vi "Add Request Form Field.vi"(8 "error in (no error)":errorcluster, 10 "FormField":refnum<class "FormField.lvclass">, 11 "Request in":refnum<class "Request.lvclass">) -> (0 "error out":errorcluster, 3 "Request out":refnum<class "Request.lvclass">)   [LabVIEW 2020, in "HTTP Utils.lvlib" / "Request.lvclass"]
uses:
  Request.lvclass
  FormField/FormField.lvclass
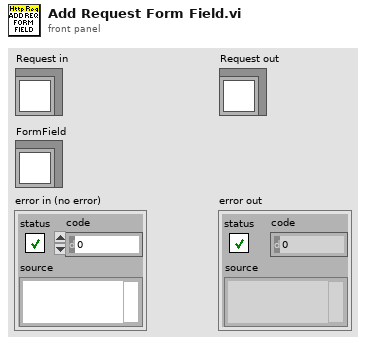
[diagram p1: front panel]
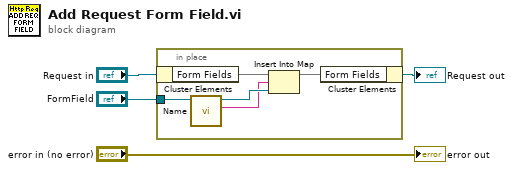
[diagram p0: block diagram]
diagram:
  n1 = in-place {
    in-place-border: "FormField" -> [w9]
    n2 = in-place-cluster #1("Request in") -> ("Form Fields"=w8:map{string, refnum<class "FormField.lvclass">})
    n3 = call "Name.vi"("FormField in"=w9) -> ("Name"=w6:string, "FormField out"=w7:refnum<class "FormField.lvclass">)  [unwired: 8 in, 1 out]
    n4 = Insert Into Map(map in=w8, key=w6, value=w7) -> (map out=w5:map{string, refnum<class "FormField.lvclass">})  [unwired: 2 out]
    n5 = in-place-cluster #1("Form Fields"=w5) -> (→"Request out":refnum<class "Request.lvclass">)
  }
  "error out" <- "error in (no error)"
